vi "Setup.vi"(9 "Active Project":refnum<vi>, 10 "NI.LV.Dialog Instance":refnum<vi>) -> (1 "Project Type Name Library File Path":T1, 2 "Target":string, 3 "_Rescript out":refnum<class "_Rescript.lvclass">, 4 "All Type Name Library File Path":T1)   [LabVIEW 2020, in "_Rescript.lvlib" / "_Rescript.lvclass"]
uses:
  _Rescript.lvclass
  _Rescript.lvclass/_Rescript.ctl
  _Shared/Project Stuff/Project Stuff.lvclass
  _Shared/Name Library File Path.ctl
  _Shared/_Shared.lvlib
  _Shared/Type.ctl
  _Shared/Type Name Library File Path.ctl
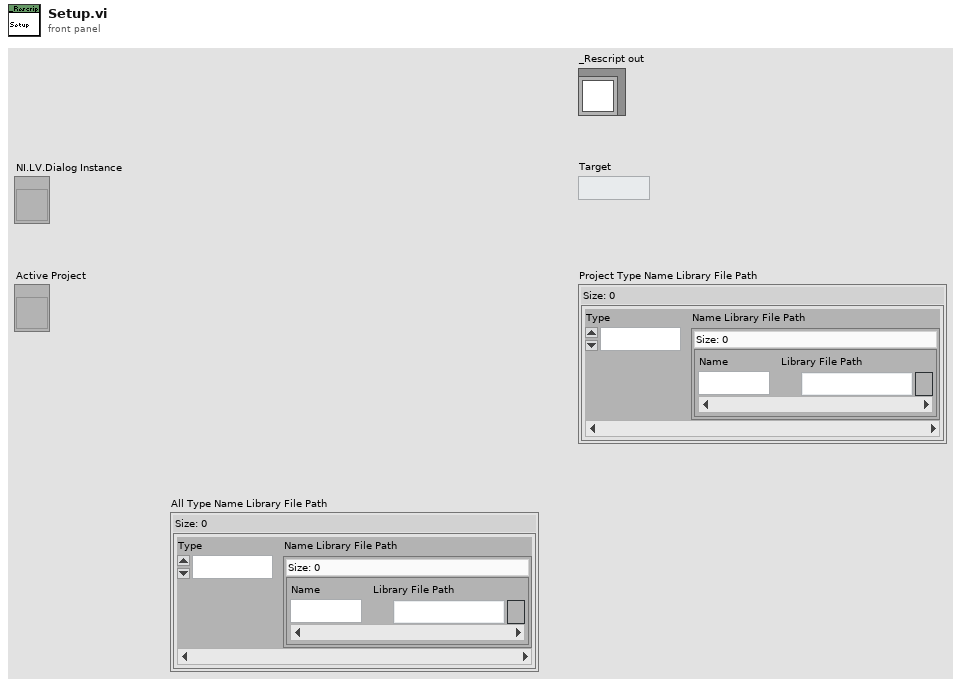
[diagram p1: front panel]
types:
  T1 = typedef "_Shared.lvlib/Type Name Library File Path.ctl" = map{T2, T3}
  T2 = typedef "_Shared.lvlib/Type.ctl" = enum16{"Actor", "Msg"}
  T3 = typedef "_Shared.lvlib/Name Library File Path.ctl" = map{string, path}
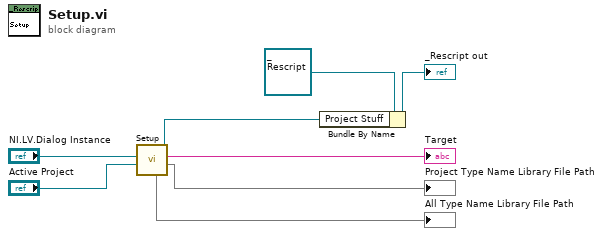
[diagram p0: block diagram]
diagram:
  n1 = call "Setup.vi"("Active Project"="Active Project", "NI.LV.Dialog Instance"="NI.LV.Dialog Instance") -> ("Project Type Name Library File Path"=→"Project Type Name Library File Path":T1, "Target"=→"Target":string, "Project Stuff out"=w4:refnum<class "Project Stuff.lvclass">, "All Type Name Library File Path"=→"All Type Name Library File Path":T1)  [unwired: 6 in]
  n2 = Bundle By Name(cluster=refnum<class "_Rescript.lvclass"> refnum ("_Rescript Msg out"), "Project Stuff"=w4) -> (→"_Rescript out":refnum<class "_Rescript.lvclass">)
